vi "Displayed Row Calc.vi"(7 "Constant Sizes":T1, 8 "Coords.Vertical":i32, 9 "Tree.Position:Top":i32, 10 "Top Left Visible Cell":T2, 11 "TreeItems":T3[](array[typedef])) -> (1 "Top left visible TreeItem index":i32, 2 "Pixels from top of row":i32, 3 "Displayed Row":i32)   [LabVIEW 2020, in "BetterDragAndDrop.lvlib" / "BetterTreeHandle.lvclass"]
uses:
  Classes/BetterTreeHandle/BetterTreeHandle.lvclass
  Classes/BetterTreeItem/SubVIs/TreeItem.ctl
  <vilib>/Utility/miscctls.llb/LVNodeAndColumnTypeDef.ctl
  Classes/BetterHandle/Pixel Constants.ctl
  BetterDragAndDrop.lvlib
  Classes/BetterHandle/BetterHandle.lvclass
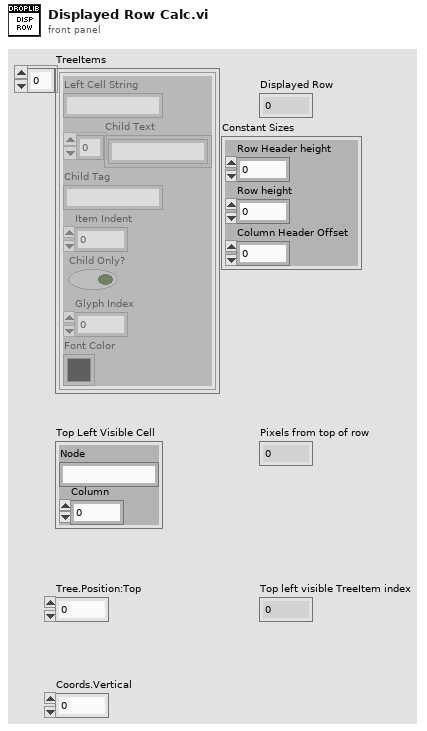
[diagram p1: front panel]
types:
  T1 = typedef "BetterDragAndDrop.lvlib/BetterHandle.lvclass/Pixel Constants.ctl" = cluster{"Row Header height":i32, "Row height":i32, "Column Header Offset":i32}
  T2 = typedef "LVNodeAndColumnTypeDef.ctl" = cluster{"Node":string, "Column":i32}
  T3 = typedef "BetterDragAndDrop.lvlib/BetterTreeHandle.lvclass/TreeItem.ctl" = cluster{"Left Cell String":string, "Child Text":string[], "Child Tag":string, "Item Indent":i32, "Child Only?":bool, "Glyph Index":i32, "Font Color":u32}
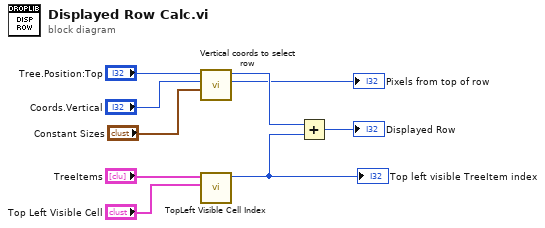
[diagram p0: block diagram]
diagram:
  n1 = call "Vertical coords to select row.vi"("Constant Sizes"="Constant Sizes", "Coords.Vertical"="Coords.Vertical", "Tree.Position:Top"="Tree.Position:Top") -> ("Pixels from top of row"=→"Pixels from top of row":i32, "Displayed Row"=w5:i32)  [unwired: 7 in]
  n2 = call "TopLeft Visible Cell Index.vi"("Top Left Visible Cell"="Top Left Visible Cell", "TreeItems"="TreeItems") -> ("TreeItem idex (Top left visible)"=w4:i32)  [unwired: 9 in]
  "Top left visible TreeItem index" <- w4
  n3 = Add(x=w5, y=w4) -> (x+y=→"Displayed Row":i32)
